vi "LeveledGaussianFit2D.vi"(0 "Coord Y":dbl[][](array[numeric]) format="%.2f", 1 "Threshold":dbl, 3 "Coord X":dbl[][](array[numeric]) format="%.2f", 4 "Image":dbl[][](array[numeric]) format="%.2f") -> (2 "Bary Y":dbl format="%.2f", 5 "Bary X":dbl format="%.2f")   [LabVIEW 2009]
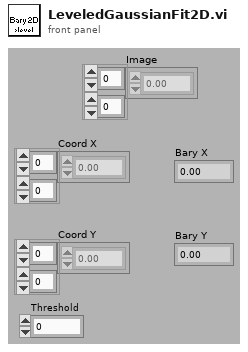
[diagram p1: front panel]
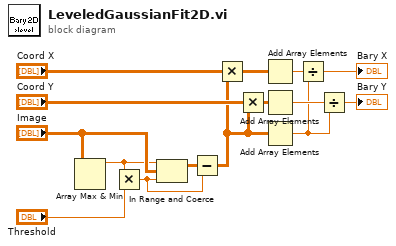
[diagram p0: block diagram]
diagram:
  n1 = Array Max & Min(array="Image") -> (max value=w4:dbl)  [unwired: 3 out]
  n2 = Multiply(x=w4, y="Threshold") -> (x*y=w2:dbl)
  n3 = In Range and Coerce(upper limit=w4, x="Image", lower limit=w2) -> (coerced(x)=w3:dbl[][])  [unwired: 1 out]
  n4 = Subtract(x=w3, y=w2) -> (x-y=w1:dbl[][])
  n5 = Multiply(x="Coord X", y=w1) -> (x*y=w11:dbl[][])
  n6 = Multiply(x="Coord Y", y=w1) -> (x*y=w10:dbl[][])
  n7 = Add Array Elements(numeric array=w11) -> (sum=w14:dbl)
  n8 = Add Array Elements(numeric array=w10) -> (sum=w9:dbl)
  n9 = Add Array Elements(numeric array=w1) -> (sum=w8:dbl)
  n10 = Divide(x=w14, y=w8) -> (x/y=→"Bary X":dbl)
  n11 = Divide(x=w9, y=w8) -> (x/y=→"Bary Y":dbl)
